vi "TESTER_v3.vi"() -> ()   [LabVIEW 2014, in "PICam.lvlib"]
uses:
  PICam.lvlib
  Ctrls/PicamROI.ctl
panel:
  in  "ReadoutTimeout":i32
  out "errors (U64/enum)":u64
  out "readout_rate (DBL)":dbl
  out "AcquisitionBuffer":i8[](array[numeric])
  out "IsAcquisitionRunning":bool
  in  "ReadoutCount":i64
  in  "Exit":bool
  in  "Stop":bool
  in  "Start":bool
  in  "ExposureTime (ms)":dbl=300.0
  out "Raw CCD data":u16[][](graph)
  out "Total pixel number":i32=132561
  in  "PicamROI":T1={"x"=1, "width"=1339, "x_binning"=1, "y"=1, "height"=99, "y_binning"=1}
  out "Frame size (bytes)":i32=265122
  out "Camera detected?":bool=TRUE
  in  "cam index":i32
  out "error out":errorcluster
  # "Less important?\n\n- Picam_DestroyString()\n- Picam_GetEnumnerationString()\n- Picam_DestroyCameraIDs()\n- Picam_GetUnavailableCameraIDs()\n+ other Destroy-methods and gettype methods"
  # "To implement:\n\n- Picam_IsLibraryInitialized()\n- Picam_IsCameraIDConnected()\n- Picam_IsCameraIDOpenElsewhere()\n- Picam_DestroyHandles()\n- Picam_GetOpenCameras()\n- Picam_IsCameraConnected()\n- Picam_IsCameraFaulted()\n- Picam_GetFirmwareDetails()\n- Picam_CanSetParameterOnline()\n- Picam_CanReadParameter() \n- Picam_CanWaitForStatusParameter()\n- Picam_GetStatusParameterPurview()\n- Picam_EstimateTimeToStatusParameterValue()\n- Picam_WaitForStatusParameterValue()\n- Picam_CommitParameters()\n- Picam_AreParametersCommited()\n- Picam_IsAcquisitionRunning()\n- Picam_WaitForAcquisitionUpdate()\n- PicamAdvanced_GetAcquisitionBuffer()\n- PicamAdvanced_SetAcquisitionBuffer()\n- PicamAdvanced_HasAcquisitionBufferOverrun()"
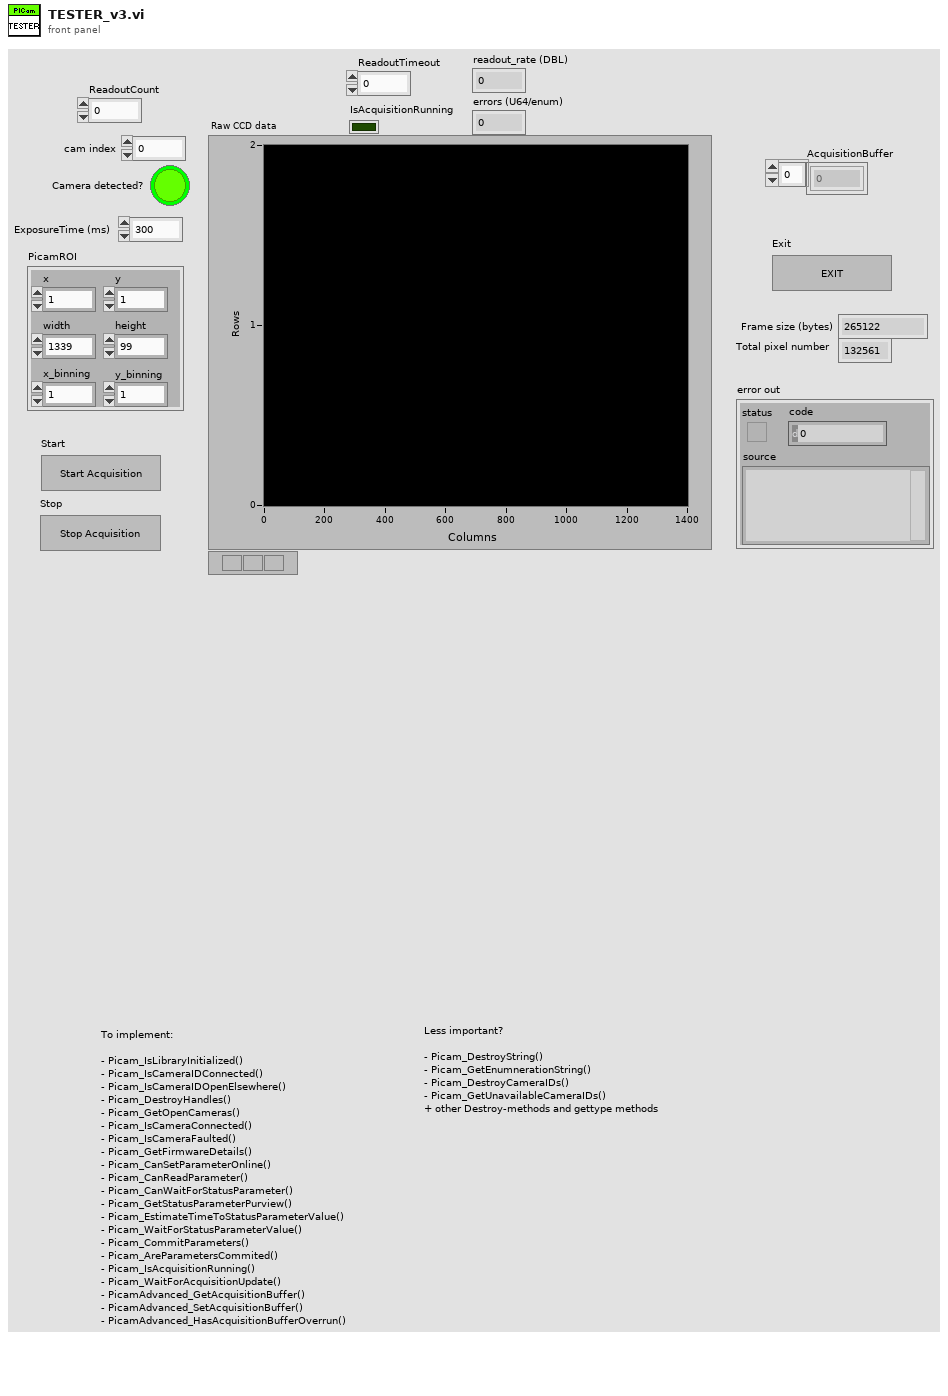
[diagram p1: front panel]
types:
  T1 = typedef "PICam.lvlib/PicamROI.ctl" = cluster{"x":i32, "width":i32, "x_binning":i32, "y":i32, "height":i32, "y_binning":i32}
  T2 = typedef "PICam.lvlib/PicamCameraID.ctl" = cluster{"PicamModel":T3, "PicamComputerInterface":T4, "sensor_name":T5, "serial_number":T6}
  T3 = typedef "PICAM.lvlib/PicamModel.ctl" = u32
  T4 = typedef "PICAM.lvlib/PicamComputerInterface.ctl" = u32
  T5 = typedef "PICAM.lvlib/sensor_name.ctl" = cluster{"U8":u8, "U8 2":u8, "U8 3":u8, "U8 4":u8, "U8 5":u8, "U8 6":u8, "U8 7":u8, "U8 8":u8, "U8 9":u8, "U8 10":u8, "U8 11":u8, "U8 12":u8, "U8 13":u8, "U8 14":u8, "U8 15":u8, "U8 16":u8, "U8 17":u8, "U8 18":u8, "U8 19":u8, "U8 20":u8, "U8 21":u8, "U8 22":u8, "U8 23":u8, "U8 24":u8, "U8 25":u8, "U8 26":u8, "U8 27":u8, "U8 28":u8, "U8 29":u8, "U8 30":u8, "U8 31":u8, "U8 32":u8, "U8 33":u8, "U8 34":u8, "U8 35":u8, "U8 36":u8, "U8 37":u8, "U8 38":u8, "U8 39":u8, "U8 40":u8, "U8 41":u8, "U8 42":u8, "U8 43":u8, "U8 44":u8, "U8 45":u8, "U8 46":u8, "U8 47":u8, "U8 48":u8, "U8 49":u8, "U8 50":u8, "U8 51":u8, "U8 52":u8, "U8 53":u8, "U8 54":u8, "U8 55":u8, "U8 56":u8, "U8 57":u8, "U8 58":u8, "U8 59":u8, "U8 60":u8, "U8 61":u8, "U8 62":u8, "U8 63":u8, "U8 64":u8}
  T6 = typedef "PICAM.lvlib/serial_number.ctl" = cluster{"U8":u8, "U8 2":u8, "U8 3":u8, "U8 4":u8, "U8 5":u8, "U8 6":u8, "U8 7":u8, "U8 8":u8, "U8 9":u8, "U8 10":u8, "U8 11":u8, "U8 12":u8, "U8 13":u8, "U8 14":u8, "U8 15":u8, "U8 16":u8, "U8 17":u8, "U8 18":u8, "U8 19":u8, "U8 20":u8, "U8 21":u8, "U8 22":u8, "U8 23":u8, "U8 24":u8, "U8 25":u8, "U8 26":u8, "U8 27":u8, "U8 28":u8, "U8 29":u8, "U8 30":u8, "U8 31":u8, "U8 32":u8, "U8 33":u8, "U8 34":u8, "U8 35":u8, "U8 36":u8, "U8 37":u8, "U8 38":u8, "U8 39":u8, "U8 40":u8, "U8 41":u8, "U8 42":u8, "U8 43":u8, "U8 44":u8, "U8 45":u8, "U8 46":u8, "U8 47":u8, "U8 48":u8, "U8 49":u8, "U8 50":u8, "U8 51":u8, "U8 52":u8, "U8 53":u8, "U8 54":u8, "U8 55":u8, "U8 56":u8, "U8 57":u8, "U8 58":u8, "U8 59":u8, "U8 60":u8, "U8 61":u8, "U8 62":u8, "U8 63":u8, "U8 64":u8}
  T7 = cluster{"running (I64/bool)":i64, "errors (U64/enum)":u64, "readout_rate (DBL)":dbl}
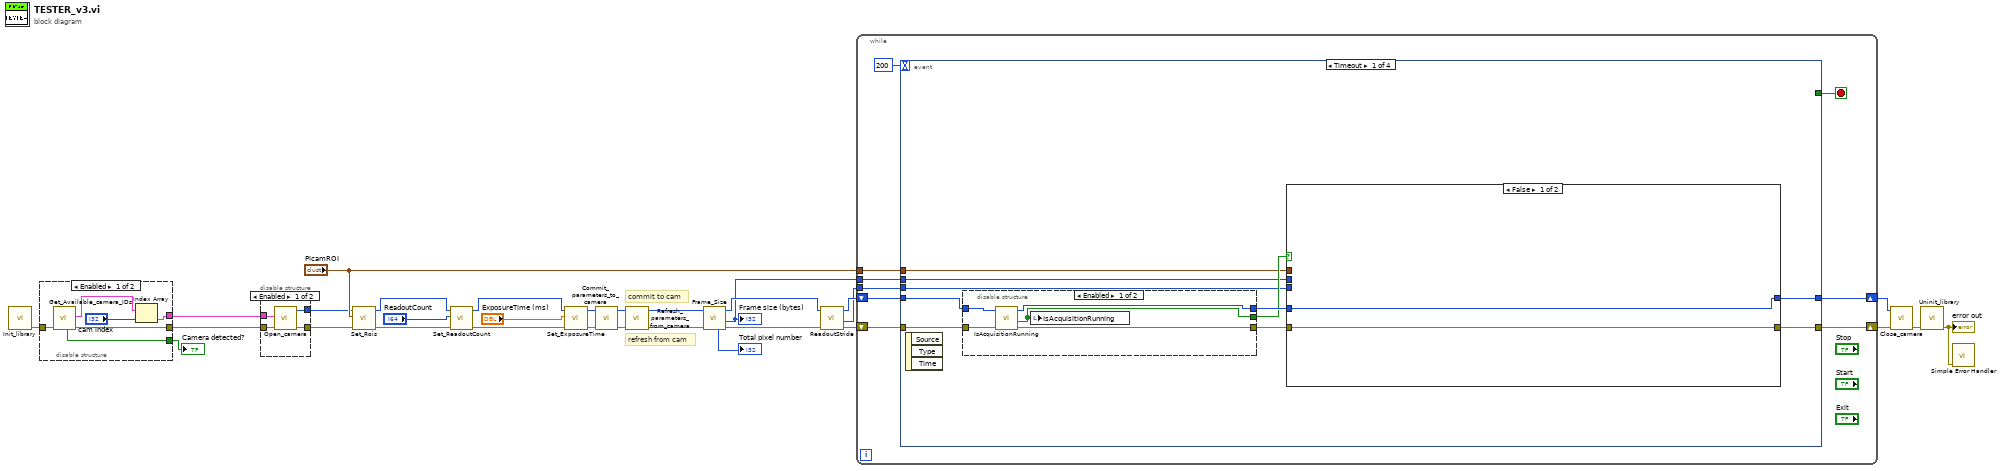
[diagram p0: block diagram]
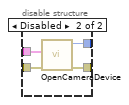
[diagram p2: hidden frame]
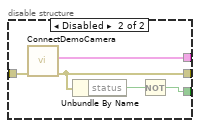
[diagram p3: hidden frame]
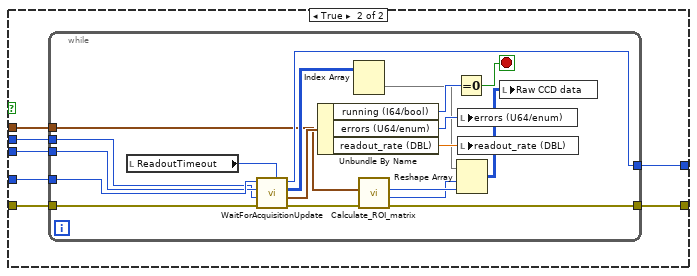
[diagram p4: hidden frame]
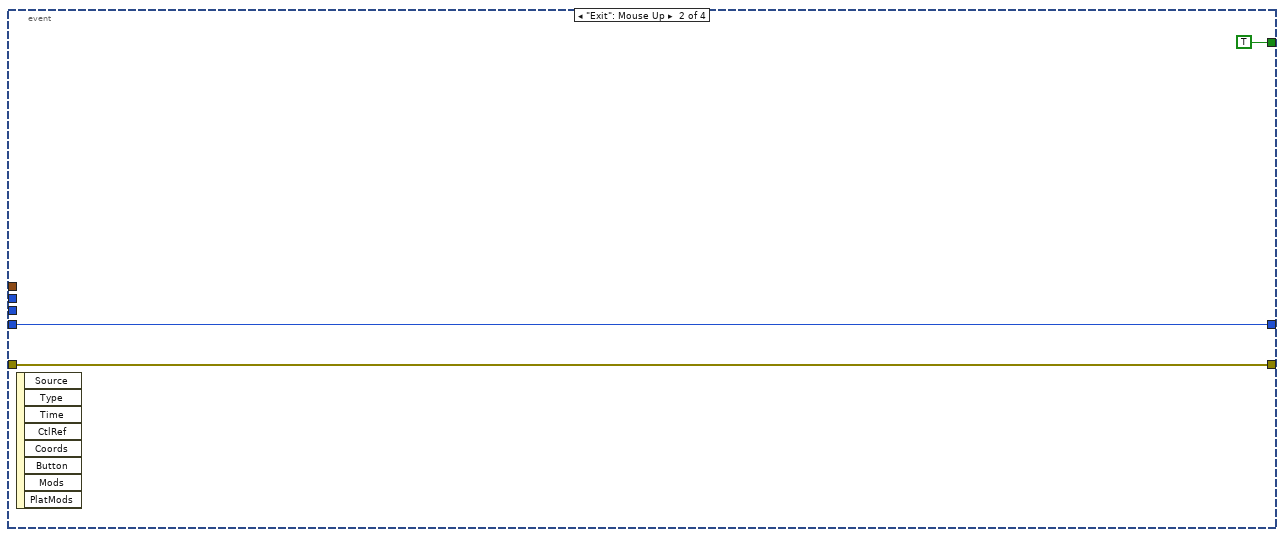
[diagram p6: hidden frame]
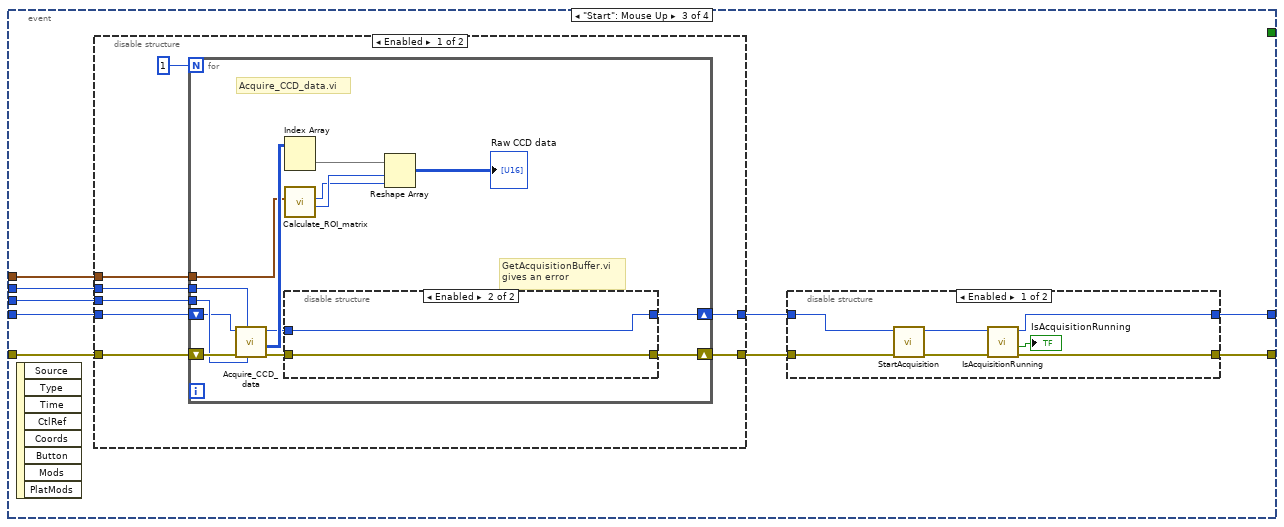
[diagram p7: hidden frame]
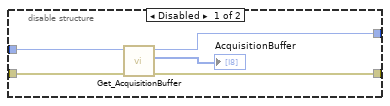
[diagram p9: hidden frame]
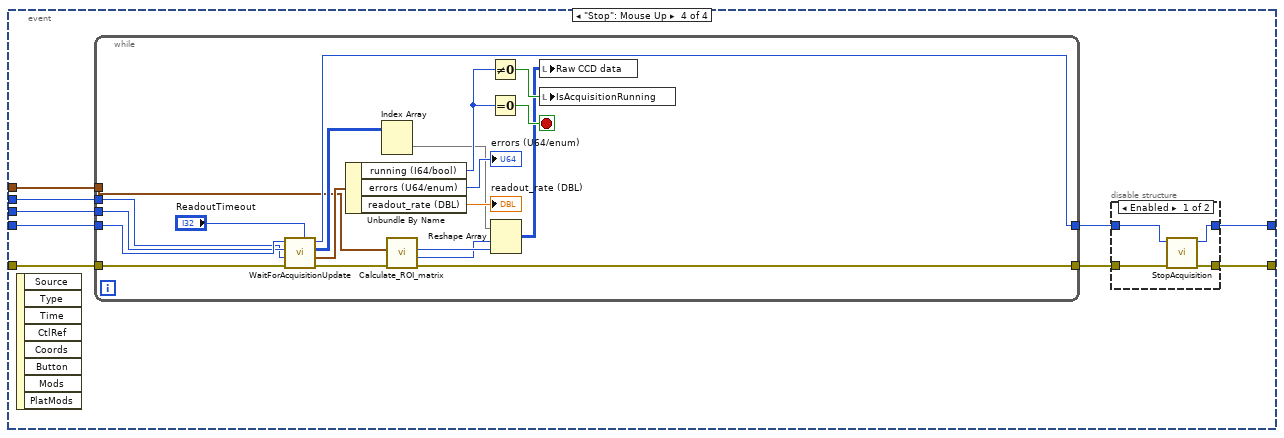
[diagram p11: hidden frame]
diagram:
  # "refresh from cam"
  # "commit to cam"
  n1 = call "Init_library.vi"() -> ("error out"=w30:errorcluster)  [unwired: 11 in]
  n2 = disable-structure shown="Enabled" {
    disable-tunnel: w30 -> [w36 w41]
    disable-tunnel: [w33 w37] -> w29
    disable-tunnel: [w32 w39] -> w2
    disable-tunnel: [w31 w40] -> w3
    frame Enabled {
      n3 = call "Get_Available_camera_IDs.vi"("error in"=w36) -> ("error out"=w32:errorcluster, "PicamCameraIDs"=w35:T2[], "Camera detected?"=w33:bool)  [unwired: 8 in]
      n4 = Index Array(array=w35, index="cam index") -> (element=w31:T2)
    }
    frame Disabled {
      n5 = call "ConnectDemoCamera.vi"("error in"=w41) -> ("error out"=w39:errorcluster, "PicamCameraID"=w40:T2)  [unwired: 8 in, 1 out]
      n6 = Unbundle By Name(w39) -> ("status"=w38:bool)
      n7 = Not(x=w38) -> (.not. x?=w37:bool)
    }
  }
  "Camera detected?" <- w29
  n8 = disable-structure shown="Enabled" {
    disable-tunnel: [w45 w46] -> w4
    disable-tunnel: w3 -> [w44 w49]
    disable-tunnel: w2 -> [w43 w48]
    disable-tunnel: [w42 w47] -> w1
    frame Enabled {
      n9 = call "Open_camera.vi"("error in"=w43, "PicamCameraID"=w44) -> ("error out"=w42:errorcluster, "camera handler out"=w45:u64)  [unwired: 8 in]
    }
    frame Disabled {
      n10 = call "OpenCameraDevice.vi"("error in"=w48, "PicamCameraID"=w49) -> ("error out"=w47:errorcluster, "camera handler out"=w46:u64)  [unwired: 8 in]
    }
  }
  n11 = call "Set_Rois.vi"("error in"=w1, "PicamROI"="PicamROI", "camera handle in"=w4) -> ("error out"=w9:errorcluster, "camera handle out"=w7:u64)  [unwired: 7 in]
  n12 = call "Set_ReadoutCount.vi"("error in"=w9, "ReadoutCount"="ReadoutCount", "camera handle in"=w7) -> ("error out"=w8:errorcluster, "camera handle out"=w6:u64)  [unwired: 7 in]
  n13 = call "Set_ExposureTime.vi"("error in"=w8, "ExposureTime (ms)"="ExposureTime (ms)", "camera handle in"=w6) -> ("error out"=w13:errorcluster, "camera handle out"=w20:u64)  [unwired: 7 in]
  n14 = call "Commit_parameters_to_camera.vi"("error in"=w13, "camera handle in"=w20) -> ("error out"=w21:errorcluster, "camera handle out"=w22:u64)  [unwired: 8 in]
  n15 = call "Refresh_parameters_from_camera.vi"("error in"=w21, "camera handle in"=w22) -> ("error out"=w18:errorcluster, "camera handle out"=w14:u64)  [unwired: 8 in]
  n16 = call "Frame_Size.vi"("error in"=w18, "camera handle in"=w14) -> ("error out"=w25:errorcluster, "Frame size (bytes)"=w16:i32, "camera handle out"=w26:u64, "Total pixel number"=→"Total pixel number":i32)  [unwired: 5 in, 1 out]
  "Frame size (bytes)" <- w16
  n17 = call "ReadoutStride.vi"("error in"=w25, "camera handle in"=w26) -> ("error out"=w23:errorcluster, "ReadoutStride (bytes)"=w15:i32, "camera handle out"=w24:u64)  [unwired: 7 in]
  n18 = while {
    tunnel: w16 -> [w56]
    tunnel: w15 -> [w55]
    tunnel: "PicamROI" -> [w52]
    shift-right: [w54] -> w12
    shift-left: w24 -> [w58]
    shift-right: [w53] -> w11
    shift-left: w23 -> [w57]
    stop <- w51 stop-if-true
    n19 = event shown="[0] Timeout" {
      selector: _ -> [_ _ _ _]
      dyn-events: _ -> [_ _ _ _]
      timeout: 200 -> [_ _ _ _]
      tunnel: w58 -> [w68 w105 w111 w162]
      tunnel: w57 -> [w67 w104 w114 w160]
      tunnel: w56 -> [w59 _ w115 w156]
      tunnel: w55 -> [w60 _ w113 w157]
      tunnel: [w64 w105 w107 w164] -> w54
      tunnel: [w63 w104 w108 w163] -> w53
      tunnel: w52 -> [w61 _ w112 w158]
      tunnel: [_ TRUE _ _] -> w51
      event Timeout {
        n20 = event-data() -> ()  [unwired: 1 in, 3 out]
        n21 = disable-structure shown="Enabled" {
          disable-tunnel: w68 -> [w101 w103]
          disable-tunnel: w67 -> [w100 w102]
          disable-tunnel: [w99 w102] -> w65
          disable-tunnel: [w98 w103] -> w66
          disable-tunnel: [w97 _] -> w62
          frame Enabled {
            n22 = call "IsAcquisitionRunning.vi"("error in"=w100, "camera handle in"=w101) -> ("error out"=w99:errorcluster, "IsAcquisitionRunning"=w97:bool, "camera handle out"=w98:u64)  [unwired: 7 in]
            n23 = local write "IsAcquisitionRunning"(w97) -> ()
          }
          frame Disabled {
          }
        }
        n24 = case shown="False" w62 {
          tunnel: w66 -> [w70 w77]
          tunnel: w65 -> [w69 w76]
          tunnel: [w70 w75] -> w64
          tunnel: [w69 w74] -> w63
          tunnel: w61 -> [_ w73]
          tunnel: w60 -> [_ w72]
          tunnel: w59 -> [_ w71]
          frame False {
          }
          frame True {
            n25 = while {
              tunnel: w77 -> [w96]
              tunnel: w76 -> [w95]
              tunnel: [w94] -> w75
              tunnel: [w82] -> w74
              tunnel: w73 -> [w84]
              tunnel: w72 -> [w79]
              tunnel: w71 -> [w78]
              stop <- w91 stop-if-true
              n26 = local read "ReadoutTimeout"() -> (w88:i32)
              n27 = call "WaitForAcquisitionUpdate.vi"("ReadoutTimeout"=w88, "error in"=w95, "frame size (bytes)"=w78, "readout_stride (bytes)"=w79, "camera handler in"=w96) -> ("error out"=w83:errorcluster, "Status"=w93:T7, "read_count * frames"=w85:u16[][], "camera handler out"=w94:u64)  [unwired: 3 in]
              n28 = Unbundle By Name(w93) -> ("running (I64/bool)"=w92:i64, "errors (U64/enum)"=w90:u64, "readout_rate (DBL)"=w89:dbl)
              n29 = Index Array(array=w85) -> (element=w87:u16[])  [unwired: 2 in]
              n30 = call "Calculate_ROI_matrix.vi"("error in (no error)"=w83, "PicamROI"=w84) -> ("error out"=w82:errorcluster, "Columns (pixels)"=w81:i32, "Rows (pixels)"=w86:i32)  [unwired: 7 in]
              n31 = Equal To 0?(x=w92) -> (x = 0?=w91:bool)
              n32 = Reshape Array(w87, w81, w86) -> (w80:u16[][])
              n33 = local write "errors (U64/enum)"(w90) -> ()
              n34 = local write "readout_rate (DBL)"(w89) -> ()
              n35 = local write "Raw CCD data"(w80) -> ()
            }
          }
        }
      }
      event "Exit": Mouse Up {
        n36 = event-data() -> ()  [unwired: 1 in, 8 out]
      }
      event "Start": Mouse Up {
        n37 = event-data() -> ()  [unwired: 1 in, 8 out]
        n38 = disable-structure shown="Enabled" {
          disable-tunnel: w115 -> [w132 _]
          disable-tunnel: w114 -> [w131 w155]
          disable-tunnel: w113 -> [w130 _]
          disable-tunnel: w112 -> [w129 _]
          disable-tunnel: w111 -> [w128 w154]
          disable-tunnel: [w126 w154] -> w110
          disable-tunnel: [w127 w155] -> w109
          frame Enabled {
            n39 = for {
              N: 1 -> [_]
              tunnel: w132 -> [w146]
              tunnel: w130 -> [w144]
              tunnel: w129 -> [w140]
              shift-right: [w136] -> w127
              shift-left: w131 -> [w145]
              shift-right: [w135] -> w126
              shift-left: w128 -> [w139]
              # "Acquire_CCD_data.vi"
              # "GetAcquisitionBuffer.vi\ngives an error"
              n40 = call "Acquire_CCD_data.vi"("readout_stride (bytes)"=w144, "frame size (bytes)"=w146, "error in"=w145, "camera handle in"=w139) -> ("error out"=w137:errorcluster, "read_count * frames"=w141:u16[][], "camera handle out"=w138:u64)  [unwired: 4 in, 1 out]
              n41 = Index Array(array=w141) -> (element=w142:u16[])  [unwired: 2 in]
              n42 = call "Calculate_ROI_matrix.vi"("PicamROI"=w140) -> ("Columns (pixels)"=w134:i32, "Rows (pixels)"=w133:i32)  [unwired: 8 in, 1 out]
              n43 = disable-structure shown="Enabled" {
                disable-tunnel: w138 -> [w151 w153]
                disable-tunnel: w137 -> [w150 w152]
                disable-tunnel: [w149 w152] -> w136
                disable-tunnel: [w148 w153] -> w135
                frame Disabled {
                  n44 = call "Get_AcquisitionBuffer.vi"("error in"=w150, "camera handler in"=w151) -> ("error out"=w149:errorcluster, "AcquisitionBuffer"=→"AcquisitionBuffer":i8[], "camera handler out"=w148:u64)  [unwired: 7 in]
                }
                frame Enabled {
                }
              }
              n45 = Reshape Array(w142, w134, w133) -> (→"Raw CCD data":u16[][])
            }
          }
          frame Disabled {
          }
        }
        n46 = disable-structure shown="Enabled" {
          disable-tunnel: w110 -> [w122 w124]
          disable-tunnel: w109 -> [w121 w123]
          disable-tunnel: [w118 w123] -> w108
          disable-tunnel: [w117 w124] -> w107
          frame Enabled {
            n47 = call "StartAcquisition.vi"("error in"=w121, "camera handle in"=w122) -> ("error out"=w119:errorcluster, "camera handle out"=w120:u64)  [unwired: 8 in]
            n48 = call "IsAcquisitionRunning.vi"("error in"=w119, "camera handle in"=w120) -> ("error out"=w118:errorcluster, "IsAcquisitionRunning"=→"IsAcquisitionRunning":bool, "camera handle out"=w117:u64)  [unwired: 7 in]
          }
          frame Disabled {
          }
        }
      }
      event "Stop": Mouse Up {
        n49 = event-data() -> ()  [unwired: 1 in, 8 out]
        n50 = while {
          tunnel: w162 -> [w184]
          tunnel: w160 -> [w183]
          tunnel: [w182] -> w161
          tunnel: [w168] -> w159
          tunnel: w158 -> [w170]
          tunnel: w157 -> [w166]
          tunnel: w156 -> [w165]
          stop <- w178 stop-if-true
          n51 = call "WaitForAcquisitionUpdate.vi"("ReadoutTimeout"="ReadoutTimeout", "error in"=w183, "frame size (bytes)"=w165, "readout_stride (bytes)"=w166, "camera handler in"=w184) -> ("error out"=w169:errorcluster, "Status"=w181:T7, "read_count * frames"=w171:u16[][], "camera handler out"=w182:u64)  [unwired: 3 in]
          n52 = Unbundle By Name(w181) -> ("running (I64/bool)"=w177:i64, "errors (U64/enum)"=→"errors (U64/enum)":u64, "readout_rate (DBL)"=→"readout_rate (DBL)":dbl)
          n53 = Index Array(array=w171) -> (element=w174:u16[])  [unwired: 2 in]
          n54 = call "Calculate_ROI_matrix.vi"("error in (no error)"=w169, "PicamROI"=w170) -> ("error out"=w168:errorcluster, "Columns (pixels)"=w172:i32, "Rows (pixels)"=w173:i32)  [unwired: 7 in]
          n55 = Not Equal To 0?(x=w177) -> (x != 0?=w176:bool)
          n56 = Equal To 0?(x=w177) -> (x = 0?=w178:bool)
          n57 = Reshape Array(w174, w172, w173) -> (w167:u16[][])
          n58 = local write "Raw CCD data"(w167) -> ()
          n59 = local write "IsAcquisitionRunning"(w176) -> ()
        }
        n60 = disable-structure shown="Enabled" {
          disable-tunnel: w161 -> [w188 w190]
          disable-tunnel: [w187 w190] -> w164
          disable-tunnel: w159 -> [w186 w189]
          disable-tunnel: [w185 w189] -> w163
          frame Enabled {
            n61 = call "StopAcquisition.vi"("error in"=w186, "camera handle in"=w188) -> ("error out"=w185:errorcluster, "camera handle out"=w187:u64)  [unwired: 8 in]
          }
          frame Disabled {
          }
        }
      }
    }
  }
  n62 = call "Close_camera.vi"("error in"=w11, "camera handle in"=w12) -> ("error out"=w28:errorcluster)  [unwired: 9 in]
  n63 = call "Uninit_library.vi"("error in"=w28) -> ("error out"=w17:errorcluster)  [unwired: 10 in]
  "error out" <- w17
  n64 = call <vilib>:"Simple Error Handler.vi"("error in (no error)"=w17) -> ()  [unwired: 4 in, 5 out]
